vi "Bridge Open.vi"(8 "error in":errorcluster, 11 "bridge in":T1={"type"=enum."TWM client", "TWM"={"pipe name"="", "parameters"=[], "handle"=0, "fixed aper [s]"=0.0, "f-list [Hz]"=[], "discrete f-list"=FALSE, "unc mode"=enum."None", "unc mcc"=0, "unc first"=FALSE}, "last f"=0.0, "bias comp"={"bias type"=enum."dummy", "VISA"="", "Enable"=FALSE, "channel qu"=[], "channel Uinit"=[]}, "sim mode"=enum."Generic RLC network", "channel idns"=[], "sim phases"=1} {"TWM"."f-list [Hz]" format="%#_6p"}) -> (0 "error out":errorcluster, 1 "bias idn string":string, 2 "idn string":string, 3 "bridge out":T1={"type"=enum."TWM client", "TWM"={"pipe name"="", "parameters"=[], "handle"=0, "fixed aper [s]"=0.0, "f-list [Hz]"=[], "discrete f-list"=FALSE, "unc mode"=enum."None", "unc mcc"=0, "unc first"=FALSE}, "last f"=0.0, "bias comp"={"bias type"=enum."dummy", "VISA"="", "Enable"=FALSE, "channel qu"=[], "channel Uinit"=[]}, "sim mode"=enum."Generic RLC network", "channel idns"=[], "sim phases"=1} {"TWM"."f-list [Hz]" format="%#_6p"})   [LabVIEW 2013]
doc: "Open and initialize bridge."
uses:
  Bridge Session.ctl
  Bridge Type.ctl
  drivers/TWM client/TWM Session.ctl
  drivers/TWM client/TWM parameters.ctl
  drivers/TWM client/Meas Proc QWTB Uncertainty Mode.ctl
  Bridge Bias Session.ctl
  Bridge Bias Type.ctl
  Bridge Sim Mode.ctl
  drivers/TWM client.lvlibp
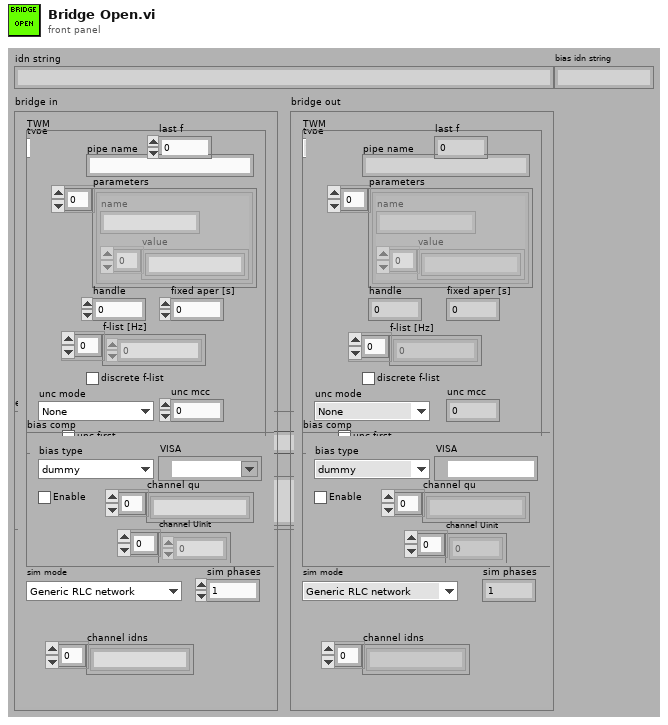
[diagram p1: front panel]
types:
  T1 = typedef "Bridge Session.ctl" = cluster{"type":T2, "TWM":T3, "last f":dbl, "bias comp":T6, "sim mode":T8, "channel idns":string[], "sim phases":i32}
  T2 = typedef "Bridge Type.ctl" = enum16{"TWM client", "dummy"}
  T3 = typedef "TWM Session.ctl" = cluster{"pipe name":string, "parameters":T4[], "handle":i32, "fixed aper [s]":dbl, "f-list [Hz]":dbl[], "discrete f-list":bool, "unc mode":T5, "unc mcc":i32, "unc first":bool}
  T4 = typedef "TWM parameters.ctl" = cluster{"name":string, "value":string[]}
  T5 = typedef "Meas Proc QWTB Uncertainty Mode.ctl" = enum16{"None", "GUF", "Monte Carlo"}
  T6 = typedef "Bridge Bias Session.ctl" = cluster{"bias type":T7, "VISA":refnum<visa-resource-name>, "Enable":bool, "channel qu":string[], "channel Uinit":dbl[]}
  T7 = typedef "Bridge Bias Type.ctl" = enum16{"dummy", "CMI LiBbias V1.0"}
  T8 = typedef "Bridge Sim Mode.ctl" = enum16{"Generic RLC network", "Interchannel transfer"}
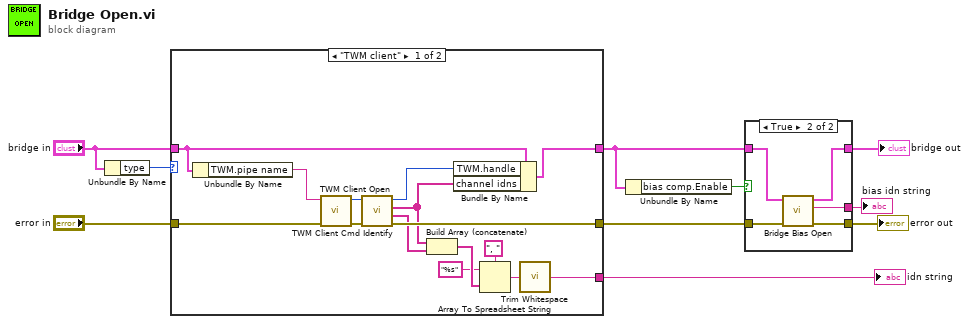
[diagram p0: block diagram]
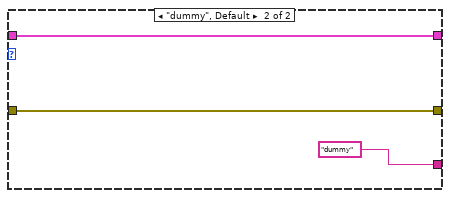
[diagram p3: hidden frame]
diagram:
  n1 = Unbundle By Name("bridge in") -> ("type"=w10:T2)
  n2 = case shown="\"TWM client\"" w10 {
    tunnel: "error in" -> [w25 w28]
    tunnel: [w19 w28] -> w6
    tunnel: "bridge in" -> [w24 w26]
    tunnel: [w18 w26] -> w3
    tunnel: [w12 "dummy"] -> w7
    frame "TWM client" {
      n3 = Unbundle By Name(w24) -> ("TWM.pipe name"=w23:string)
      n4 = call "TWM Client Open.vi"("error in"=w25, "pipe name"=w23) -> ("error out"=w22:errorcluster, "handle out"=w21:i32)  [unwired: 8 in]
      n5 = call "TWM Client Cmd Identify.vi"("error in"=w22, "handle"=w21) -> ("error out"=w19:errorcluster, "aux idns"=w17:string[], "channel idns"=w11:string[], "handle out"=w20:i32)  [unwired: 6 in]
      n6 = Build Array (concatenate)(w11, w17) -> (w16:string[])
      n7 = Bundle By Name(cluster=w24, "TWM.handle"=w20, "channel idns"=w11) -> (w18:T1)
      n8 = Array To Spreadsheet String(delimiter (Tab)=", ", array=w16, 3:"%s" ("format string")) -> (spreadsheet string=w13:string)
      n9 = call <vilib>:"Trim Whitespace.vi"("string"=w13) -> ("trimmed string"=w12:string)  [unwired: 1 in]
    }
    frame "dummy", Default {
    }
  }
  "idn string" <- w7
  n10 = Unbundle By Name(w3) -> ("bias comp.Enable"=w4:bool)
  n11 = case shown="True" w4 {
    tunnel: w6 -> [w29 w35]
    tunnel: [w29 w34] -> w5
    tunnel: w3 -> [w30 w33]
    tunnel: [w30 w32] -> w2
    tunnel: [_ w31] -> w1
    frame False {
    }
    frame True {
      n12 = call "Bridge Bias Open.vi"("error in"=w35, "bridge in"=w33) -> ("error out"=w34:errorcluster, "idn string"=w31:string, "bridge out"=w32:T1)  [unwired: 7 in]
    }
  }
  "error out" <- w5
  "bridge out" <- w2
  "bias idn string" <- w1
